vi "Search By Selection.vi"(0 "App Refnum":refnum<vi>, 1 "Project Item Names":string[](array[string])=["Parrent.lvclass [My Computer< Untitled Project 1.lvproj]", "Child.lvclass [My Computer< Untitled Project 1.lvproj]", "QD Test.vi [My Computer< Untitled Project 1.lvproj]", "Find Project Items.vi [QuickDrop< My Computer< Untitled Project 1.lvproj]", "Get Default QD Object Shortcuts File.vi [QuickDrop< My Computer< Untitled Project 1.lvproj]", "Load Default QD Object Shortcuts.vi [QuickDrop< My Computer< Untitled Project 1.lvproj]", "OldSearchAlgorithm.vi [QuickDrop< My Computer< Untitled Project 1.lvproj]", "OpenSearchWrapper.vi [QuickDrop< My Computer< Untitled Project 1.lvproj]", "QuickDrop Get QDKS Info for Shortcut Dialog.vi [QuickDrop< My Computer< Untitled Project 1.lvproj]", "QuickDrop Get QDKS Mappings.vi [QuickDrop< My Computer< Untitled Project 1.lvproj]", "QuickDrop Get Shortcut Info.vi [QuickDrop< My Computer< Untitled Project 1.lvproj]", "QuickDrop Get Terminal Names.vi [QuickDrop< My Computer< Untitled Project 1.lvproj]", "QuickDrop Get Wire Prefix.vi [QuickDrop< My Computer< Untitled Project 1.lvproj]", "QuickDrop Launch Window.vi [QuickDrop< My Computer< Untitled Project 1.lvproj]", "QuickDrop Get Wire Query terms.vi [QuickDrop< My Computer< Untitled Project 1.lvproj]", "QuickDrop Insert String into Array.vi [QuickDrop< My Computer< Untitled Project 1.lvproj]", "QuickDrop Plugin Template.vit [QuickDrop< My Computer< Untitled Project 1.lvproj]", "QuickDrop Populate QDKS Listbox.vi [QuickDrop< My Computer< Untitled Project 1.lvproj]", "QuickDrop Process Drop Information.vi [QuickDrop< My Computer< Untitled Project 1.lvproj]", "QuickDrop QDKS Info.ctl [QuickDrop< My Computer< Untitled Project 1.lvproj]", "QuickDrop Read QDKS INI Info.vi [QuickDrop< My Computer< Untitled Project 1.lvproj]", "QuickDrop Shortcut Config.vi [QuickDrop< My Computer< Untitled Project 1.lvproj]", "QuickDrop Get Wire Class Query terms.vi [QuickDrop< My Computer< Untitled Project 1.lvproj]", "Parrent_Create.vi [Parrent.lvclass< My Computer< Untitled Project 1.lvproj]", "Destroy.vi [Parrent.lvclass< My Computer< Untitled Project 1.lvproj]", "Child_Create.vi [Child.lvclass< My Computer< Untitled Project 1.lvproj]", "Destroy.vi [Child.lvclass< My Computer< Untitled Project 1.lvproj]", "Method 1.vi [Child.lvclass< My Computer< Untitled Project 1.lvproj]", "Method 2.vi [Child.lvclass< My Computer< Untitled Project 1.lvproj]", "LV Config Read.vi [Dependencies< My Computer< Untitled Project 1.lvproj]", "LV Config Read Boolean.vi [Dependencies< My Computer< Untitled Project 1.lvproj]", "LV Config Read String.vi [Dependencies< My Computer< Untitled Project 1.lvproj]", "LV Config Read Pathlist.vi [Dependencies< My Computer< Untitled Project 1.lvproj]", "LV Config Read Color.vi [Dependencies< My Computer< Untitled Project 1.lvproj]", "LV Config Read Numeric (I32).vi [Dependencies< My Computer< Untitled Project 1.lvproj]", "LV Config Write.vi [Dependencies< My Computer< Untitled Project 1.lvproj]", "LV Config Write Boolean.vi [Dependencies< My Computer< Untitled Project 1.lvproj]", "LV Config Write String.vi [Dependencies< My Computer< Untitled Project 1.lvproj]", "LV Config Write Pathlist.vi [Dependencies< My Computer< Untitled Project 1.lvproj]", "LV Config Write Color.vi [Dependencies< My Computer< Untitled Project 1.lvproj]", "LV Config Write Numeric (I32).vi [Dependencies< My Computer< Untitled Project 1.lvproj]", "VSI TSVN Tbar_SVN Lock with Dialog.vi [Dependencies< My Computer< Untitled Project 1.lvproj]", "VSI TSVN Tbar_Handle SVN Error.vi [Dependencies< My Computer< Untitled Project 1.lvproj]", "Status Dialog Display Button.vi [Dependencies< My Computer< Untitled Project 1.lvproj]", "Status Dialog Justify Text.vi [Dependencies< My Computer< Untitled Project 1.lvproj]", "Status Dialog Update Message.vi [Dependencies< My Computer< Untitled Project 1.lvproj]", "Status Dialog Exit.vi [Dependencies< My Computer< Untitled Project 1.lvproj]", "Status Dialog Init.vi [Dependencies< My Computer< Untitled Project 1.lvproj]", "Status Dialog Wait for Status Queue.vi [Dependencies< My Computer< Untitled Project 1.lvproj]", "Status Dialog.vi [Dependencies< My Computer< Untitled Project 1.lvproj]", "Insert.vi [plugins< QuickDrop< My Computer< Untitled Project 1.lvproj]", "Move Labels.vi [plugins< QuickDrop< My Computer< Untitled Project 1.lvproj]", "Remove and Rewire.vi [plugins< QuickDrop< My Computer< Untitled Project 1.lvproj]", "Replace.vi [plugins< QuickDrop< My Computer< Untitled Project 1.lvproj]", "SVN Commit.vi [plugins< QuickDrop< My Computer< Untitled Project 1.lvproj]", "SVN Lock.vi [plugins< QuickDrop< My Computer< Untitled Project 1.lvproj]", "SVN Update.vi [plugins< QuickDrop< My Computer< Untitled Project 1.lvproj]", "VI Server Rename.vi [plugins< QuickDrop< My Computer< Untitled Project 1.lvproj]", "Wire All Terminals.vi [plugins< QuickDrop< My Computer< Untitled Project 1.lvproj]", "Wire Multiple Objects Together.vi [plugins< QuickDrop< My Computer< Untitled Project 1.lvproj]", "ObjectAttributes.ctl [protected< Parrent.lvclass< My Computer< Untitled Project 1.lvproj]", "Parrent_New.vi [utils< Parrent.lvclass< My Computer< Untitled Project 1.lvproj]", "Parrent_GetAttributes.vi [utils< Parrent.lvclass< My Computer< Untitled Project 1.lvproj]", "ObjectAttributes.ctl [protected< Child.lvclass< My Computer< Untitled Project 1.lvproj]", "Child_New.vi [utils< Child.lvclass< My Computer< Untitled Project 1.lvproj]", "Child_GetAttributes.vi [utils< Child.lvclass< My Computer< Untitled Project 1.lvproj]", "TTK_FTW-ERR-CallChain.vi [TTK_FTW.lvlib< Dependencies< My Computer< Untitled Project 1.lvproj]", "TTK_FTW-ERR-Clear.vi [TTK_FTW.lvlib< Dependencies< My Computer< Untitled Project 1.lvproj]", "TTK_FTW-ERR-NoErrorConstant.vi [TTK_FTW.lvlib< Dependencies< My Computer< Untitled Project 1.lvproj]", "TTK_FTW-ERR-ThrowError.vi [TTK_FTW.lvlib< Dependencies< My Computer< Untitled Project 1.lvproj]", "TTK_FTW-Regex-ReplaceAll.vi [TTK_FTW.lvlib< Dependencies< My Computer< Untitled Project 1.lvproj]", "TTK_FTW-Regex.vi [TTK_FTW.lvlib< Dependencies< My Computer< Untitled Project 1.lvproj]", "TTK_FTW-STR-Array-Delimit.vi [TTK_FTW.lvlib< Dependencies< My Computer< Untitled Project 1.lvproj]", "TTK_FTW-STR-ReplaceWhitespace.vi [TTK_FTW.lvlib< Dependencies< My Computer< Untitled Project 1.lvproj]", "Available Non-Node.ctl [_WireMultipleSupport< plugins< QuickDrop< My Computer< Untitled Project 1.lvproj]", "Change Tunnel Modes to Fix Wires.vi [_WireMultipleSupport< plugins< QuickDrop< My Computer< Untitled Project 1.lvproj]", "Connect Valid Terminals.vi [_WireMultipleSupport< plugins< QuickDrop< My Computer< Untitled Project 1.lvproj]", "Connector Pane Position.ctl [_WireMultipleSupport< plugins< QuickDrop< My Computer< Untitled Project 1.lvproj]", "Find Top and Error Terminals.vi [_WireMultipleSupport< plugins< QuickDrop< My Computer< Untitled Project 1.lvproj]", "Get Wirable Objects from Selection.vi [_WireMultipleSupport< plugins< QuickDrop< My Computer< Untitled Project 1.lvproj]", "Group Selection List By Row.vi [_WireMultipleSupport< plugins< QuickDrop< My Computer< Untitled Project 1.lvproj]", "Match Relaxed Data Type.vi [_WireMultipleSupport< plugins< QuickDrop< My Computer< Untitled Project 1.lvproj]", "Match Source and Sink Terminals.vi [_WireMultipleSupport< plugins< QuickDrop< My Computer< Untitled Project 1.lvproj]", "Node Terminal Info.ctl [_WireMultipleSupport< plugins< QuickDrop< My Computer< Untitled Project 1.lvproj]", "Node-Terminal Pair.ctl [_WireMultipleSupport< plugins< QuickDrop< My Computer< Untitled Project 1.lvproj]", "Prepare to Wire Two Nodes.vi [_WireMultipleSupport< plugins< QuickDrop< My Computer< Untitled Project 1.lvproj]", "Sort Node Terminals.vi [_WireMultipleSupport< plugins< QuickDrop< My Computer< Untitled Project 1.lvproj]", "Sort Unwired Terminals.vi [_WireMultipleSupport< plugins< QuickDrop< My Computer< Untitled Project 1.lvproj]", "What to Wire.ctl [_WireMultipleSupport< plugins< QuickDrop< My Computer< Untitled Project 1.lvproj]", "Wire Non-Nodes to Nodes.vi [_WireMultipleSupport< plugins< QuickDrop< My Computer< Untitled Project 1.lvproj]"], 2 "Project Item Refs":refnum<vi>[](array[refnum]), 7 "VI":string, 11 "error in (no error)":errorcluster) -> (4 "Class Item Names":string[](array[string]), 8 "Query terms":string[](array[string]), 15 "error out":errorcluster)   [LabVIEW 2018]
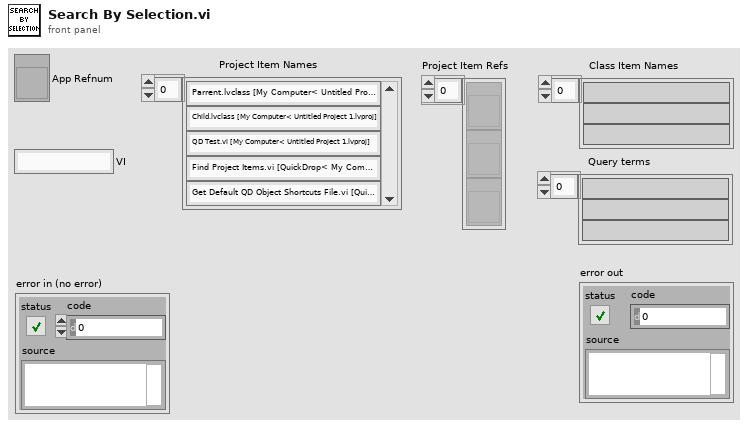
[diagram p1: front panel]
types:
  T1 = typedef "NI_Data Type.lvlib/Data Type.ctl" = enum8{"Invalid Type", "Void", "I8", "I16", "I32", "I64", "U8", "U16", "U32", "U64", "Single Float", "Double Float", "Extended Float", "Single Complex", "Double Complex", "Extended Complex", "Enum U8", "Enum U16", "Enum U32", "Enum U64", "Single Float With Unit", "Double Float With Unit", "Extended Float With Unit", "Single Complex with Unit", "Double Complex with Unit", "Extended Complex with Unit", "Boolean", "String", "Path", "Picture", "Tag", "Array", "Cluster", "Variant", "LV Variant", "Waveform", "Timestamp", "Digital Waveform", "Digital Data", "ExpressData", "Refnum", "External Data", "VI", "Poly VI", "LabVIEW Class Instance", "Fixed Point", "Set Collection", "Map Collection"}
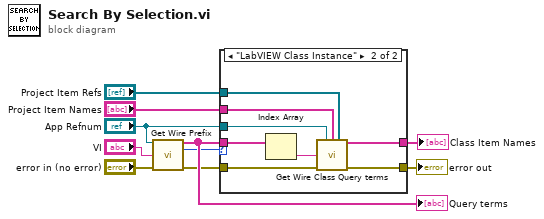
[diagram p0: block diagram]
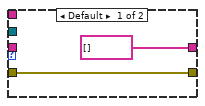
[diagram p2: hidden frame]
diagram:
  n1 = call "Get Wire Prefix.vi"("App Refnum"="App Refnum", "VI"="VI", "error in (no error)"="error in (no error)") -> ("Query terms"=w9:string[], "labVIEW Type"=w8:T1, "error out"=w3:errorcluster)  [unwired: 10 in]
  "Query terms" <- w9
  n2 = case shown="\"LabVIEW Class Instance\"" w8 {
    tunnel: w9 -> [_ w20]
    tunnel: [string[] [] ("Class Item Names") w18] -> w7
    tunnel: "App Refnum" -> [_ w17]
    tunnel: "Project Item Names" -> [_ w16]
    tunnel: "Project Item Refs" -> [_ w15]
    tunnel: w3 -> [w11 w14]
    tunnel: [w11 w13] -> w1
    frame Default {
    }
    frame "LabVIEW Class Instance" {
      n3 = Index Array(array=w20) -> (element=w19:string)  [unwired: 1 in]
      n4 = call "Get Wire Class Query terms.vi"("App Refnum"=w17, "Project Item Names"=w16, "Project Item Refs"=w15, "Class/vi name"=w19, "error in (no error)"=w14) -> ("Class Item Names"=w18:string[], "error out"=w13:errorcluster)  [unwired: 9 in]
    }
  }
  "Class Item Names" <- w7
  "error out" <- w1
